vi "count line-feed char.vi"(0 "string":string) -> ()   [LabVIEW 2013]
uses:
  mMc param - global.vi
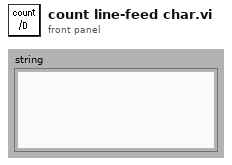
[diagram p1: front panel]
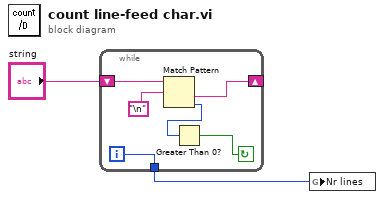
[diagram p0: block diagram]
diagram:
  n1 = while {
    shift-right: [w6] -> _
    shift-left: "string" -> [w7]
    tunnel: [w3] -> w1
    i -> [w3]
    stop <- w4 continue-if-true
    n2 = Match Pattern(string=w7, regular expression="\n") -> (after substring=w6:string, offset past match=w5:i32)  [unwired: 1 in, 2 out]
    n3 = Greater Than 0?(x=w5) -> (x > 0?=w4:bool)
  }
  n4 = global write "mMc param - global.vi" "Nr lines"(w1) -> ()
